vi "apply modification.vi"(10 "vis":refnum<vi>[](array[refnum]), 11 "execution settings in":refnum<class "execution settings.lvclass">) -> (0 "error report":errorcluster[](array[cluster]), 3 "execution settings out":refnum<class "execution settings.lvclass">)   [LabVIEW 2013, in "execution settings.lvclass"]
uses:
  execution settings.lvclass
  execution settings.lvclass/execution settings.ctl
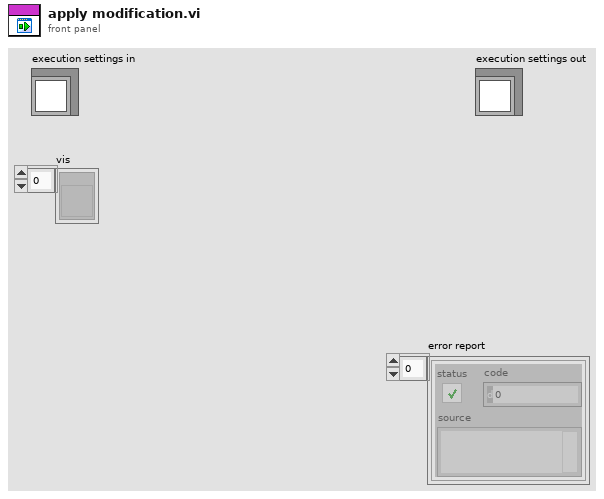
[diagram p1: front panel]
types:
  T1 = enum16{"Share clones between instances", "Preallocate clone for each instance"}
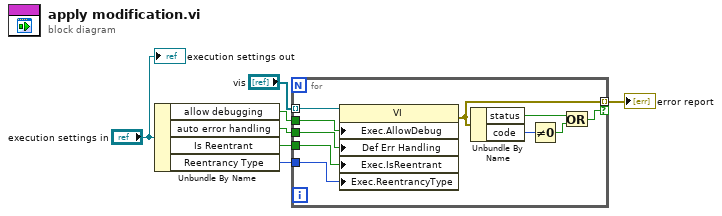
[diagram p0: block diagram]
diagram:
  n1 = Unbundle By Name("execution settings in") -> ("allow debugging"=w4:bool, "auto error handling"=w3:bool, "Is Reentrant"=w2:bool, "Reentrancy Type"=w1:T1)
  n2 = for {
    tunnel: "vis" -> [w17] mode=indexing
    tunnel: [w13] -> w6 mode=indexing if=w12
    tunnel: w4 -> [w11]
    tunnel: w3 -> [w10]
    tunnel: w2 -> [w9]
    tunnel: w1 -> [w8]
    n3 = property class="VI"(reference=w17, "Exec.AllowDebug"=w11, "Def Err Handling"=w10, "Exec.IsReentrant"=w9, "Exec.ReentrancyType"=w8) -> (error out=w13:errorcluster)  [unwired: 1 in, 1 out]
    n4 = Unbundle By Name(w13) -> ("status"=w16:bool, "code"=w15:i32)
    n5 = Not Equal To 0?(x=w15) -> (x != 0?=w14:bool)
    n6 = Or(x=w16, y=w14) -> (x .or. y?=w12:bool)
  }
  "error report" <- w6
  "execution settings out" <- "execution settings in"
